vi "Get Save Versions.vi"(8 "error in":errorcluster) -> (0 "error out":errorcluster, 2 "Test Versions":string[](array[string]))   [LabVIEW 2020, in "Library Icon Data.lvclass"]
doc: "Gets a list of versions the library can be saved in."
uses:
  Library Icon Data.lvclass
  Library Icon Data.lvclass/Library Icon Data.ctl
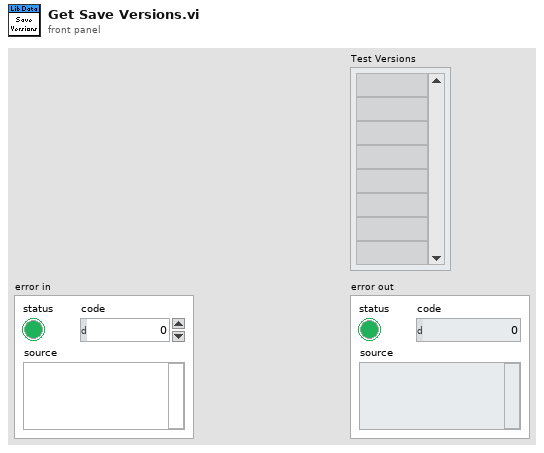
[diagram p1: front panel]
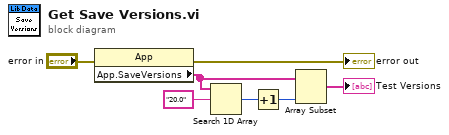
[diagram p0: block diagram]
diagram:
  n1 = property class="App"(error in="error in") -> (error out=→"error out":errorcluster, "App.SaveVersions"=w3:string[])  [unwired: 1 in, 1 out]
  n2 = Search 1D Array(1D array=w3, element="20.0" ("y")) -> (index of element=w2:i32)  [unwired: 1 in]
  n3 = Increment(x=w2) -> (x+1=w1:i32)
  n4 = Array Subset(array=w3, length=w1) -> (→"Test Versions":string[])  [unwired: 1 in]
